vi "Word_borders_shading_(adv).vi"(0 "Range in":refnum<k7>, 7 "Borders and shading":T1={"OutsideLineStyle"=0, "OutsideLineColorIndex"=4278190080, "OutsideLineWidth"=2, "BackgroundPatternColor"=4278190080} {"OutsideLineWidth" items=["wdLineWidth025pt"=2, "wdLineWidth050pt"=4, "wdLineWidth075pt"=6, "wdLineWidth100pt"=8, "wdLineWidth150pt"=12, "wdLineWidth225pt"=18, "wdLineWidth300pt"=24, "wdLineWidth450pt"=36, "wdLineWidth600pt"=48]; "OutsideLineStyle" items=["wdLineStyleNone", "wdLineStyleSingle", "wdLineStyleDot", "wdLineStyleDashSmallGap", "wdLineStyleDashLargeGap", "wdLineStyleDashDot", "wdLineStyleDashDotDot", "wdLineStyleDouble", "wdLineStyleTriple", "wdLineStyleThinThickSmallGap", "wdLineStyleThickThinSmallGap", "wdLineStyleThinThickThinSmallGap", "wdLineStyleThinThickMedGap", "wdLineStyleThickThinMedGap", "wdLineStyleThinThickThinMedGap", "wdLineStyleThinThickLargeGap", "wdLineStyleThickThinLargeGap", "wdLineStyleThinThickThinLargeGap", "wdLineStyleSingleWavy", "wdLineStyleDoubleWavy", "wdLineStyleDashDotStroked", "wdLineStyleEmboss3D", "wdLineStyleEngrave3D", "wdLineStyleOutset", "wdLineStyleInset"]}, 11 "Error in":errorcluster) -> (4 "Range out":refnum<k7>, 15 "Error out":errorcluster)   [LabVIEW 2020, in "NI_ReportGenerationToolkit.lvlib"]
uses:
  <vilib>/addons/_office/NI_ReportGenerationToolkit.lvlib
panel:
  # "Borders"
  # "Shading"
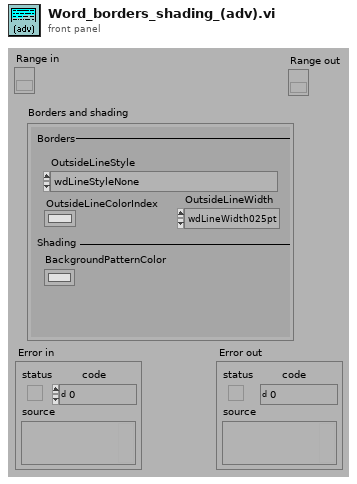
[diagram p1: front panel]
types:
  T1 = cluster{"OutsideLineStyle":i32, "OutsideLineColorIndex":u32, "OutsideLineWidth":i32, "BackgroundPatternColor":u32}
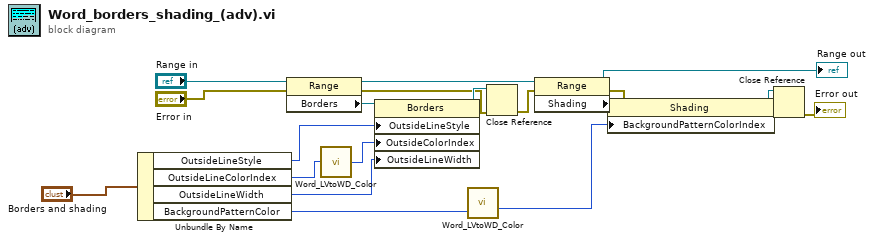
[diagram p0: block diagram]
diagram:
  n1 = Unbundle By Name("Borders and shading") -> ("OutsideLineStyle"=w7:i32, "OutsideLineColorIndex"=w4:u32, "OutsideLineWidth"=w6:i32, "BackgroundPatternColor"=w2:u32)
  n2 = property class="Range"(reference="Range in", error in="Error in") -> (reference out=w17:refnum<k7>, error out=w5:errorcluster, "Borders"=w19:refnum<k7>)
  n3 = call <vilib>:"Word_LVtoWD_Color.vi"("LabVIEW color"=w4) -> ("word color table index"=w3:i32)
  n4 = property class="Borders"(reference=w19, "OutsideLineStyle"=w7, "OutsideColorIndex"=w3, "OutsideLineWidth"=w6) -> (reference out=w13:refnum<k7>)  [unwired: 1 in, 1 out]
  n5 = call <vilib>:"Word_LVtoWD_Color.vi"("LabVIEW color"=w2) -> ("word color table index"=w1:i32)
  n6 = Close Reference(reference=w13, error in (no error)=w5) -> (error out=w11:errorcluster)
  n7 = property class="Range"(reference=w17, error in=w11) -> (reference out=→"Range out":refnum<k7>, error out=w10:errorcluster, "Shading"=w16:refnum<k7>)
  n8 = property class="Shading"(reference=w16, error in=w10, "BackgroundPatternColorIndex"=w1) -> (reference out=w14:refnum<k7>, error out=w9:errorcluster)
  n9 = Close Reference(reference=w14, error in (no error)=w9) -> (error out=→"Error out":errorcluster)
